vi "settingParamOsc (SubVI).vi"(10 "Volt":dbl, 11 "UNDT_Pulse":dbl) -> (2 "Array":T1(array[cluster]), 3 "Time":T2)   [LabVIEW 2017]
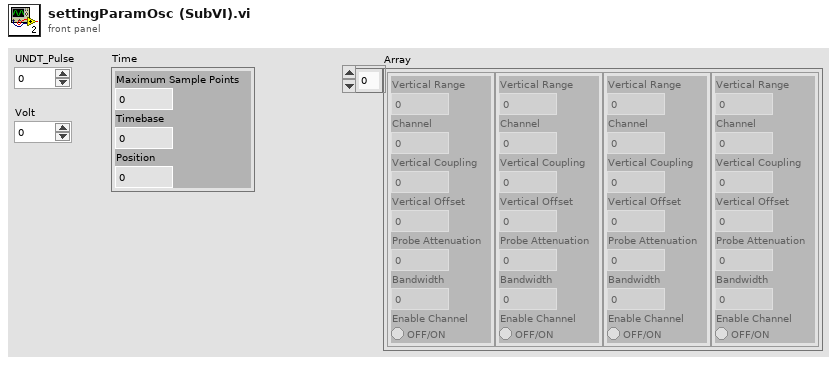
[diagram p1: front panel]
types:
  T1 = cluster{"Vertical Range":dbl, "Channel":u16, "Vertical Coupling":u16, "Vertical Offset":dbl, "Probe Attenuation":dbl, "Bandwidth":u16, "Enable Channel":bool}[]
  T2 = cluster{"Maximum Sample Points":i32, "Timebase":dbl, "Position":dbl}
  T3 = cluster{"Vertical Range":dbl, "Channel":u16, "Vertical Coupling":u16, "Vertical Offset":dbl, "Probe Attenuation":dbl, "Bandwidth":u16, "Enable Channel":bool}
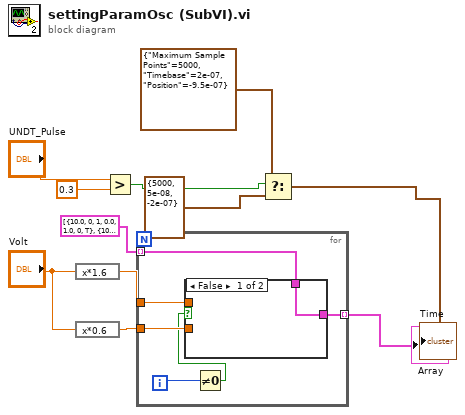
[diagram p0: block diagram]
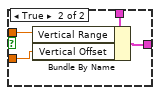
[diagram p2: hidden frame]
diagram:
  n1 = expression code="x*1.6"("Volt") -> (w3:dbl)
  n2 = expression code="x*0.6"("Volt") -> (w5:dbl)
  n3 = Greater?(x="UNDT_Pulse", y=0.3) -> (0:w10:bool)
  n4 = for {
    tunnel: T1 [{"Vertical Range"=10.0, "Channel"=0, "Vertical Coupling"=1, "Vertical Offset"=0.0, "Probe Attenuation"=1.0, "Bandwidth"=0, "Enable Channel"=TRUE}, {"Vertical Range"=10.0, "Channel"=1, "Vertical Coupling"=1, "Vertical Offset"=0.0, "Probe Attenuation"=-1.0, "Bandwidth"=0, "Enable Channel"=FALSE}, {"Vertical Range"=64.0, "Channel"=2, "Vertical Coupling"=1, "Vertical Offset"=24.0, "Probe Attenuation"=-1.0, "Bandwidth"=0, "Enable Channel"=TRUE}, {"Vertical Range"=260.0, "Channel"=3, "Vertical Coupling"=1, "Vertical Offset"=100.0, "Probe Attenuation"=-1.0, "Bandwidth"=0, "Enable Channel"=TRUE}] ("Channel config") -> [w17] mode=indexing
    tunnel: [w16] -> w2 mode=indexing
    tunnel: w3 -> [w15]
    tunnel: w5 -> [w14]
    i -> [w13]
    n5 = Not Equal To 0?(x=w13) -> (x != 0?=w12:bool)
    n6 = case shown="False" w12 {
      tunnel: w17 -> [w18 w22]
      tunnel: [w18 w21] -> w16
      tunnel: w15 -> [_ w20]
      tunnel: w14 -> [_ w19]
      frame False {
      }
      frame True {
        n7 = Bundle By Name(cluster=w22, "Vertical Range"=w20, "Vertical Offset"=w19) -> (w21:T3)
      }
    }
  }
  "Array" <- w2
  n8 = Select(t=T2 {"Maximum Sample Points"=5000, "Timebase"=2e-07, "Position"=-9.5e-07} ("Time"), s=w10, f=T2 {"Maximum Sample Points"=5000, "Timebase"=5e-08, "Position"=-2e-07} ("Time")) -> (s? t:f=→"Time":T2)
